vi "New Image Notification.vi"(8 "error in (no error)":errorcluster, 10 "Analyze Msg":refnum<class "Analyze Msg.lvclass">, 11 "Analyze Actor in":refnum<class "Analyze Actor.lvclass">) -> (0 "error out":errorcluster, 3 "Analyze Actor out":refnum<class "Analyze Actor.lvclass">)   [LabVIEW 2020]
uses:
  Analyze Actor.lvclass
  Analyze Actor Messages/Analyze Msg/Analyze Msg.lvclass
  Analyze Actor.lvclass/Analyze Actor.ctl
  C:/Program Files (x86)/National Instruments/LabVIEW 2020/vi.lib/ActorFramework/Actor/Actor.lvclass
  C:/Users/AlexK/work/LabVIEW Programme/POLARIS-AS-3-Cams/Submodules/HIJ Vision/Analyze/Analyze Actor/Analyze Actor/Analyze Actor.lvclass
  Analyze Classes/Analyze BaseClass/Analyze BaseClass/Analyze BaseClass.lvclass
  C:/Users/AlexK/work/LabVIEW Programme/POLARIS-AS-3-Cams/Submodules/HIJ Vision/Analyze/Analyze Classes/Analyze BaseClass/Analyze BaseClass/Analyze BaseClass.lvclass
  Results and Overlays/Results Base/Analyze Results Base.lvclass
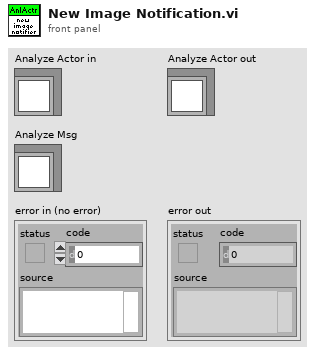
[diagram p1: front panel]
types:
  T1 = typedef "IMAQ Image.ctl" = refnum<image>
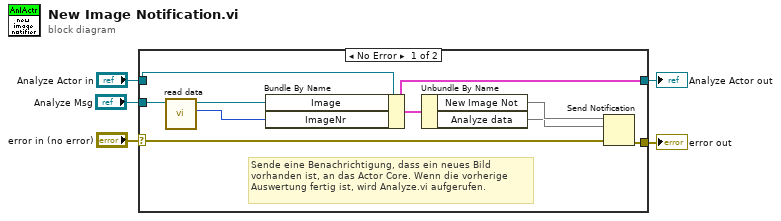
[diagram p0: block diagram]
diagram:
  n1 = case shown="No Error" "error in (no error)" {
    selector: "error in (no error)" -> [w11 w16]
    tunnel: [w10 w16] -> w4
    tunnel: [w6 w15] -> w2
    tunnel: "Analyze Actor in" -> [w7 w15]
    tunnel: "Analyze Msg" -> [w14 _]
    frame No Error {
      # "Sende eine Benachrichtigung, dass ein neues Bild\nvorhanden ist, an das Actor Core. Wenn die vorherige\nAuswertung fertig ist, wird Analyze.vi aufgerufen."
      n2 = call "read data.vi"("Analyze Msg in"=w14) -> ("Image Nr."=w12:i32, "Image"=w13:T1)  [unwired: 9 in]
      n3 = Bundle By Name(cluster=w7, "Image"=w13, "ImageNr"=w12) -> (w6:cluster{})
      n4 = Unbundle By Name(w6) -> ("New Image Not"=w9, "Analyze data"=w8)
      n5 = Send Notification(notification=w8, notifier=w9, error in (no error)=w11) -> (error out=w10:errorcluster)  [unwired: 1 out]
    }
    frame Error {
    }
  }
  "error out" <- w4
  "Analyze Actor out" <- w2
